vi "Get Item From Index.vi"(8 "error in (no error)":errorcluster caption="错误输入（无错误）", 9 "数值":i32, 11 "雇员名录管理 输入":refnum<class "雇员名录管理.lvclass"> caption="DNL_LabVIEW Object in") -> (0 "error out":errorcluster caption="错误输出", 1 "迭代器.lvlib:雇员.lvclass":refnum<class "雇员.lvclass">, 3 "雇员名录管理 输出":refnum<class "雇员名录管理.lvclass"> caption="DNL_LabVIEW Object out")   [LabVIEW 2011, in "迭代器.lvlib" / "雇员名录管理.lvclass"]
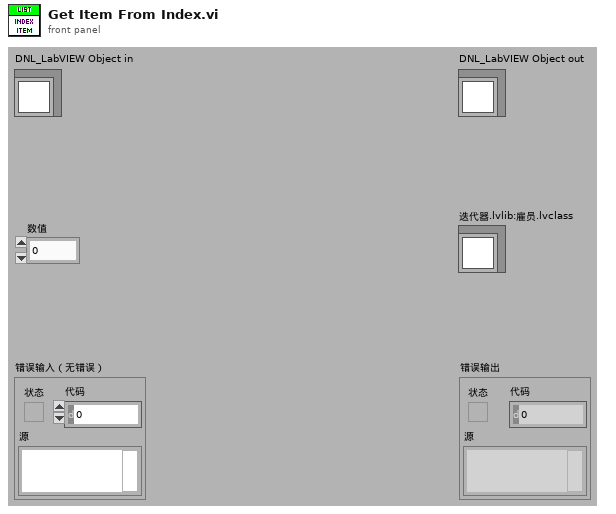
[diagram p1: front panel]
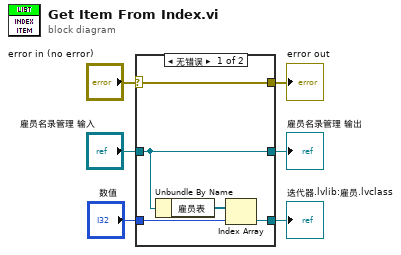
[diagram p0: block diagram]
diagram:
  n1 = case shown="无错误" "error in (no error)" {
    selector: "error in (no error)" -> [w11 w13]
    tunnel: [w11 w13] -> w5
    tunnel: [w10 w12] -> w3
    tunnel: "雇员名录管理 输入" -> [w10 w12]
    tunnel: "数值" -> [w8 _]
    tunnel: [w7 _] -> w1
    frame No Error {
      n2 = Unbundle By Name(w10) -> ("雇员表"=w9:refnum<class "雇员.lvclass">[])
      n3 = Index Array(array=w9, index=w8) -> (element=w7:refnum<class "雇员.lvclass">)
    }
    frame Error {
    }
  }
  "error out" <- w5
  "雇员名录管理 输出" <- w3
  "迭代器.lvlib:雇员.lvclass" <- w1
